vi "Interlock 32T Network Client.vi"() -> ()   [LabVIEW 2019]
doc: "Author: Scott Hannahs <sth@magnet.fsu.edu>\nCopyright 2018 Florida State University, All rights reserved."
uses:
  Interlock/SubVI/RT System Auth Level.ctl
  Interlock/SubVI/PS Action Control.ctl
  Interlock/SubVI/Interlock RT FPGA Status Info.ctl
  Interlock/SubVI/Interlock 32T FPGA Configure Parameters.ctl
  SubVIs/Interlock 32T Net Client Globals.vi
  TCP Functions/TCP Read Length and Value (STR).vi
  TCP Functions/TCP Read Length and Value (Array Str).vi
  <vilib>/Utility/miscctls.llb/LVRectTypeDef.ctl
  <vilib>/Utility/miscctls.llb/LVPointTypeDef.ctl
panel:
  in  "Clear Quench":bool
  in  "Slew rate [T/min]":dbl format="%.3g"
  out "Field [T]":dbl format="%.6g"
  in  "Setpoint [T]":dbl format="%.6g"
  in  "PS Action":T1=enum."Item 1"
  out "Version":string
  in  "Clear error":bool
  in  "Front Panel Tab":T2(tab)
  out "Crowbar Unlock Safe Curr LED":bool
  out "Crowbar":bool
  out "Quench Loop HI=ON":bool
  out "Crowbar LED":bool
  out "Close Switchbox 2":bool
  out "LTS Crowbar Status":bool
  out "HTS Crowbar Status":bool
  out "Crowbar Unlock Key":bool
  out "Ramp to Zero Button":bool
  out "Ramp to Zero Reset Button":bool
  out "Switchbox 2 Interlock":bool
  out "Switchbox 1 Interlock":bool
  out "LHe Level 2":dbl format="%.1f"
  out "LHe Level 1":dbl format="%.1f"
  out "Currents":dbl[][](graph)
  out "LHe Level":dbl[](array[slide]) scale=0.0..100.0
  out "Crowbar Unlock Gauge":dbl(knob) scale=0.0..60.0
  out "RT0 Fault Loop Timers":i16[](array[numeric])
  out "Secondary QD Time Constant":enum16{"2000 mS", "1000 mS", "200 mS", "50 mS"}(ring)
  out "HTS LEM Current":dbl format="%.5f"
  out "LTS LEM Current":dbl format="%.5f"
  out "HTS Shunt Current":dbl format="%.5f"
  out "Battery Ground Resistor V":dbl format="%.3f"
  out "Switchbox 2 Contator Out":dbl format="%.3f"
  out "Switchbox 1 Contator Out":dbl format="%.3f"
  out "Battery Voltage":dbl format="%.3f"
  out "Battery Monitory Alarm":bool
  out "Protection Logic Power Alarm":fxp<+/-,24,5> format="%.3g"
  out "Interlock RT Fault Counter":i16
  in  "Ramp To Zero Loop Time (mSec)":u32=40
  in  "PS-Disconnect Check Loop Time (mSec)":u32=40
  in  "Client Loop Time (mS)":u32=1000
  in  "Battery Low Warn":dbl format="%.1f"
  in  "Trip Threshold Currents":i16[](array[numeric])=[0, 50, 50]
  in  "Battery Voltage Scale":dbl=200.0
  in  "SW1 Vout Thresh":dbl=15.0
  in  "Quench Loop Thresh":dbl=1.5
  in  "# Low Readings":u32=3
  in  "Helium Low Level":dbl=3.0 format="%#_21g"
  in  "HTS LEM Scale":dbl=200.0
  in  "HTS Shunt Scale":dbl=40.0
  in  "LTS LEM Scale":dbl=360.0
  in  "Crowbar Loop Time (mSec)":u32=1
  in  "Interlock Check Loop Time (mSec)":u32=40
  in  "Main Loop Time (mSec)":u32=40
  in  "Turn Contactor OFF Current":dbl=1.0 format="%#_21g"
  in  "Turn Contactor ON Current":dbl=3.0 format="%#_21g"
  out "Start DateStamp":timestamp format="%<%H:%M:%S%4u\n%Y/%m/%d>T"
  out "Version RT System":string
  out "Version FPGA":string
  in  "Password":string
  in  "Save FPGA Config":bool
  in  "Read FPGA Config":bool
  out "Authorized":T3
  in  "HTS Shunt Offset (V)":dbl=40.0 format="%.4f"
  out "Download Progress":u8(slide) scale=0.0..100.0
  in  "File List":i32(listbox)=-1
  out "# Clients":u32
  out "# Timeout Err":u32
  out "Chassis Temperature":fxp<+/-,16,14> format="%.2g"
  out "Error Out":errorcluster
  in  "stop":bool
  # "NHMFL 32T\nInterlock"
  # "Indicators"
  # "Helium Levels"
  # "Coil Currents"
  # "Switch Box Status"
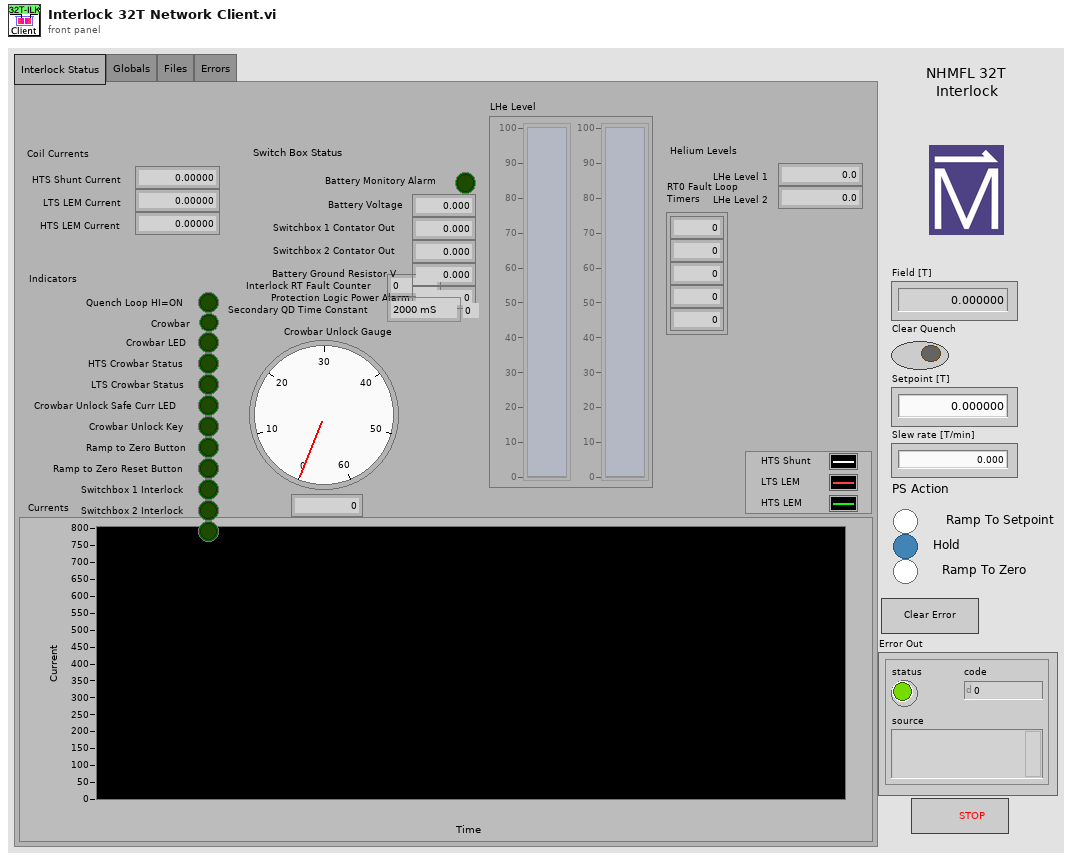
[diagram p1: front panel]
types:
  T1 = typedef "PS Action Control.ctl" = enum32{"Item 0", "Item 1", "Ramp To Zero"}
  T2 = enum32{"Interlock Status", "Globals", "Files", "Errors"}
  T3 = typedef "RT System Auth Level.ctl" = enum16{"Read Only", "User", "Operator", "Admin"}
  T4 = enum8{"Enabled", "Disabled", "Disabled and Grayed Out"}
  T5 = typedef "LVPointTypeDef.ctl" = cluster{"Horizontal":i16, "Vertical":i16}
  T6 = typedef "LVRectTypeDef.ctl" = cluster{"Left":i16, "Top":i16, "Right":i16, "Bottom":i16}
  T7 = enum16{"Standard", "Buffered", "CRLF", "Immediate"}
  T8 = typedef "Interlock 32T FPGA Configure Parameters.ctl" = cluster{"HTS LEM Scale":fxp<+/-,12,10>, "HTS Shunt Scale":fxp<+/-,16,14>, "LTS LEM Scale":fxp<+/-,12,10>, "Crowbar Loop Time (mSec)":u32, "Interlock Check Loop Time (mSec)":u32, "Main Loop Time (mSec)":u32, "Trip Threshold Currents":i16[], "Turn Contactor OFF Current":fxp<+/-,24,5>, "Turn Contactor ON Current":fxp<+/-,24,5>, "Helium Low Levels":dbl, "Quench Loop Thresh":fxp<+/-,24,5>, "SW1 Vout Thresh":fxp<+/-,24,5>, "Battery Voltage Scale":fxp<+/-,12,10>, "Battery Low Warn":dbl, "HTS Shunt Offset (V)":fxp<+/-,16,1>, "# Low Readings":u32, "PS-Disconnect Loop Time (mSec) ":u32, "Ramp To Zero Loop Time (mSec)":u32}
  T9 = typedef "Interlock RT FPGA Status Info.ctl" = cluster{"Authorized":T3, "# Clients":u32, "Chassis Temperature":fxp<+/-,16,14>, "Ramp To Zero":bool, "Crowbar":bool, "HTS Shunt":fxp<+/-,28,10>, "HTS LEM":fxp<+/-,36,15>, "LTS LEM":fxp<+/-,28,10>, "0 Reset Rt0 Button":bool, "2 Switchbox 2 Interlock":bool, "3 Switchbox 1 Interlock":bool, "5 Crowbar Unlock Safe Current LED":bool, "7 Crowbar LED":bool, "8 Ramp to Zero Button":bool, "13 Crowbar Unlock Key":bool, "15 Close Switch Box 2 Contactor":bool, "19 Battery monitor Alarm":bool, "Secondary QD Time Constant":enum16{"2000 mS", "1000 mS", "200 mS", "50 mS"}, "Loop timers":i16[], "Crowbar Latch State":i8, "Crowbar Reset Countdown Length (ms)":i32, "Crowbar Reset Countdown":i32, "Protection Petting Fault Counter":i16, "Watchdog Petting":bool, "Ramp to Zero Loop Fault Counter":i16, "Crowbar Loop Fault Counter":i16, "Main Loop Fault Counter":i16, "Interlock Petting":bool, "LTS Crowbar Status":bool, "HTS Crowbar Status":bool, "Battery Voltage":fxp<+/-,24,11>, "Protection Logic Power Alarm":fxp<+/-,24,5>, "Switchbox 2 Contactor Out":fxp<+/-,24,5>, "Battery ground resistor V":fxp<+/-,24,5>, "Switchbox 1 Contactor Out":fxp<+/-,24,5>, "Quench Loop":fxp<+/-,24,5>, "Quench Loop OK LED":bool, "10 Interlock RT Fault Counter":i16, "LHe Level 2":dbl, "LHe Level 1":dbl}
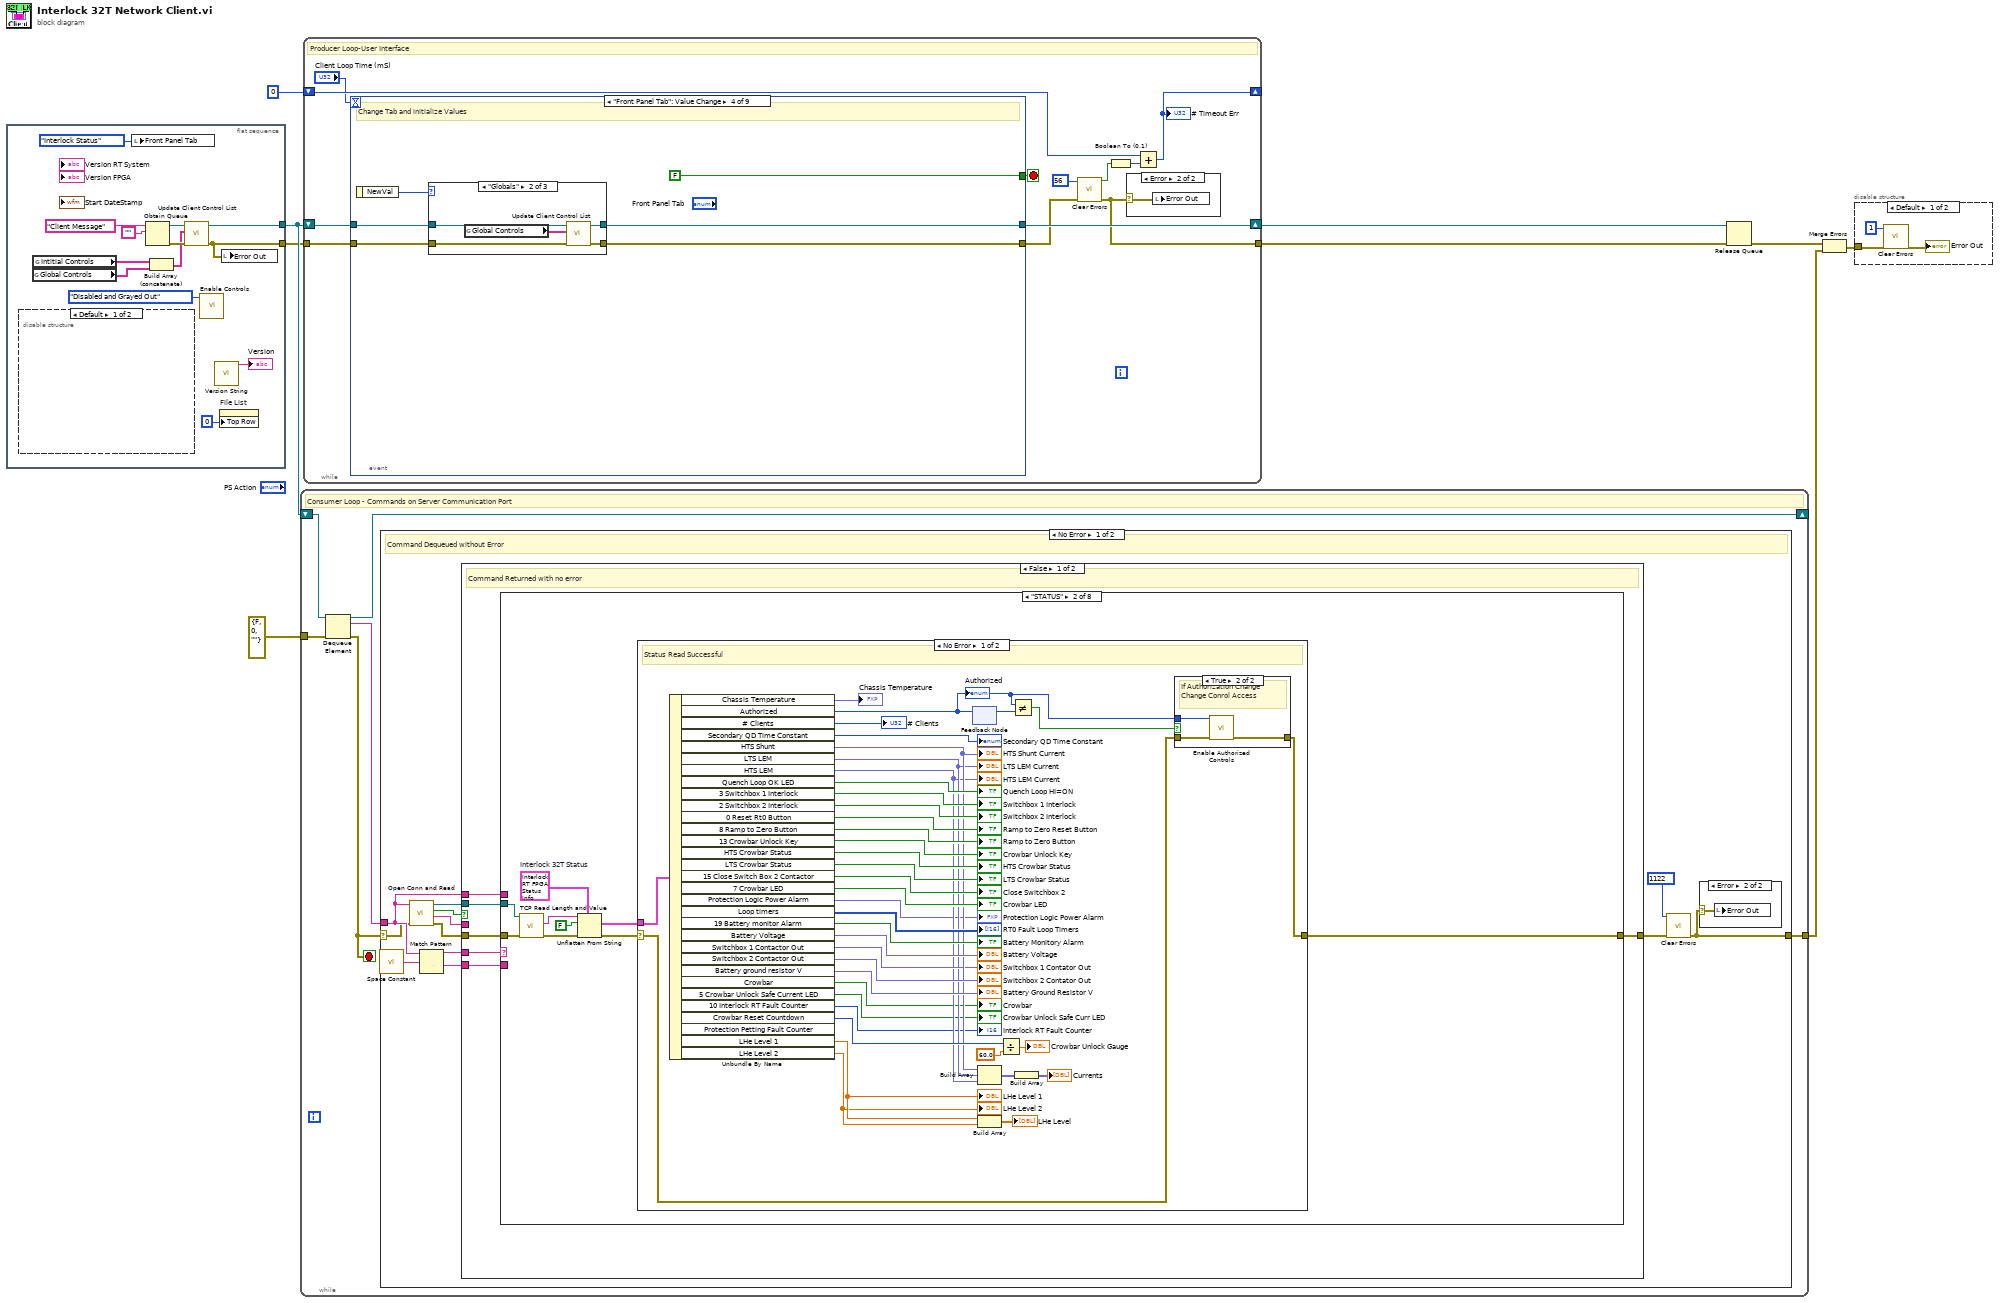
[diagram p0: block diagram]
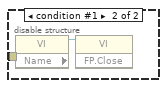
[diagram p2: hidden frame]
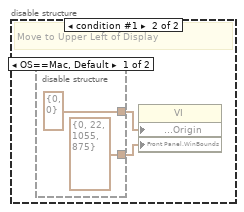
[diagram p3: hidden frame]
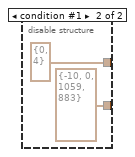
[diagram p4: hidden frame]
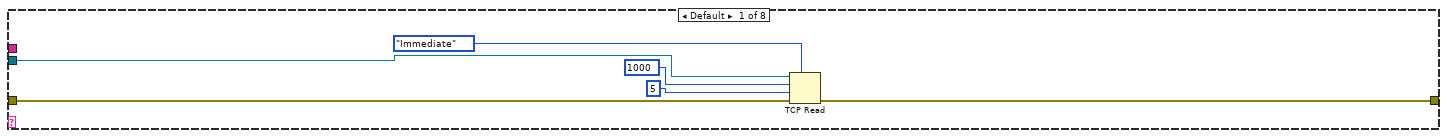
[diagram p6: hidden frame]
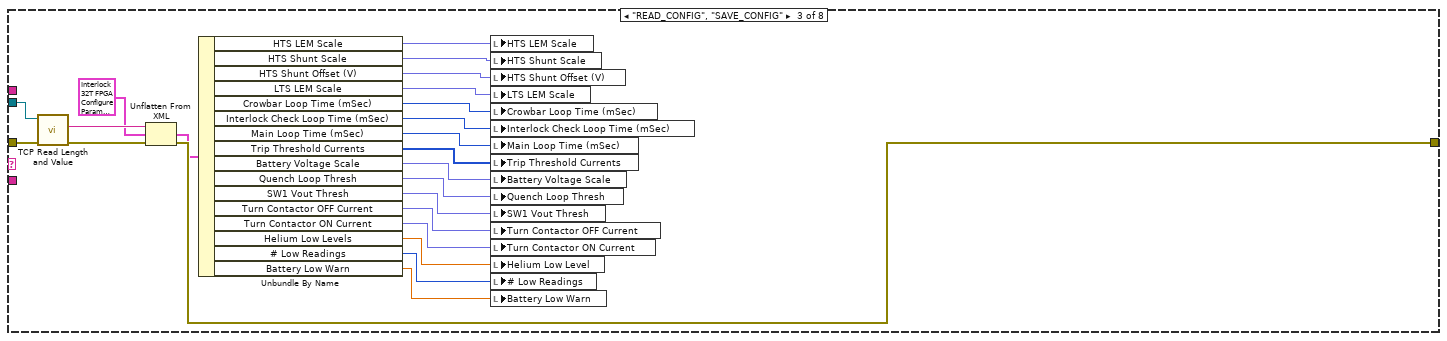
[diagram p9: hidden frame]
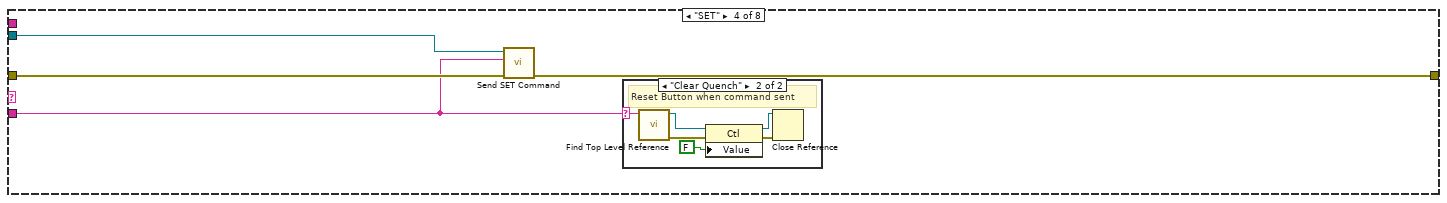
[diagram p10: hidden frame]
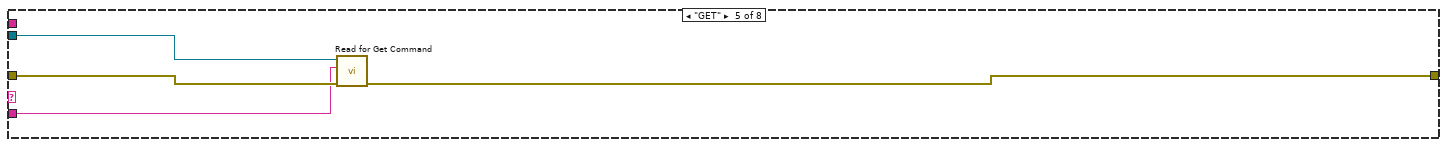
[diagram p12: hidden frame]
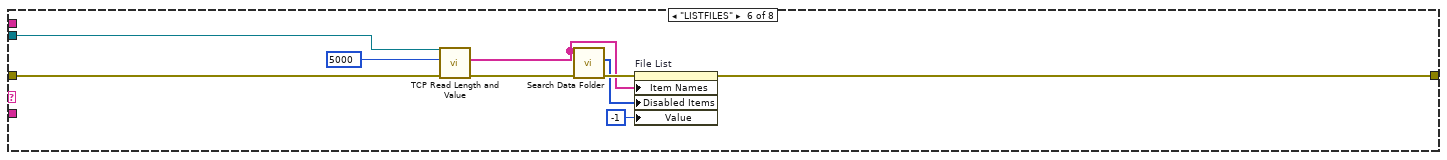
[diagram p13: hidden frame]
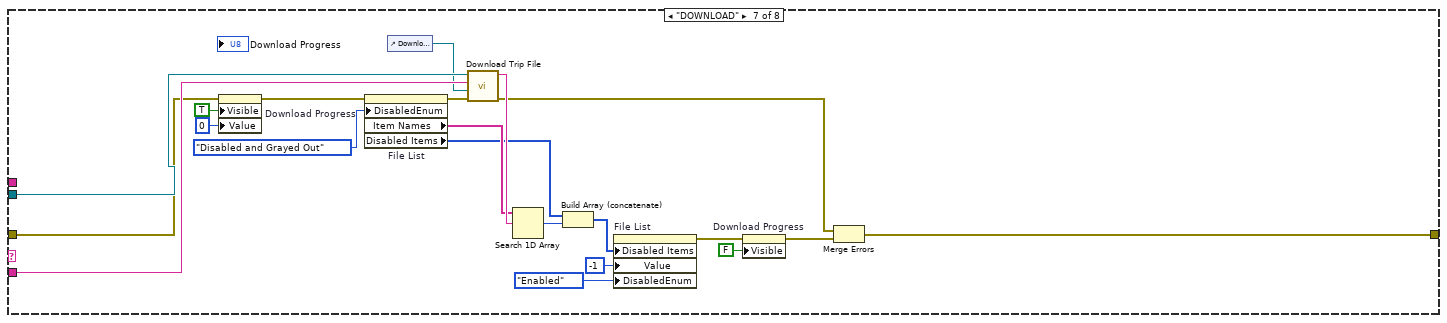
[diagram p14: hidden frame]
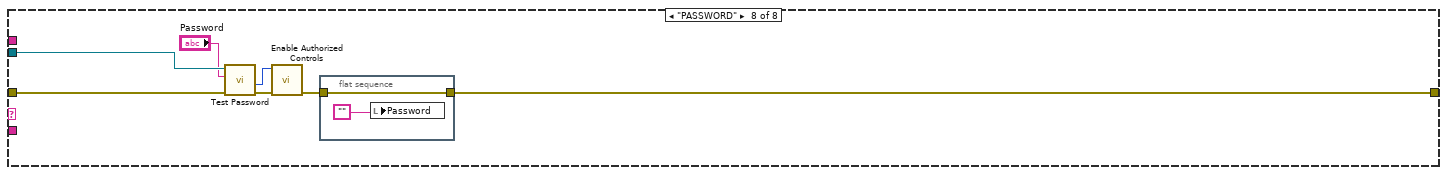
[diagram p15: hidden frame]
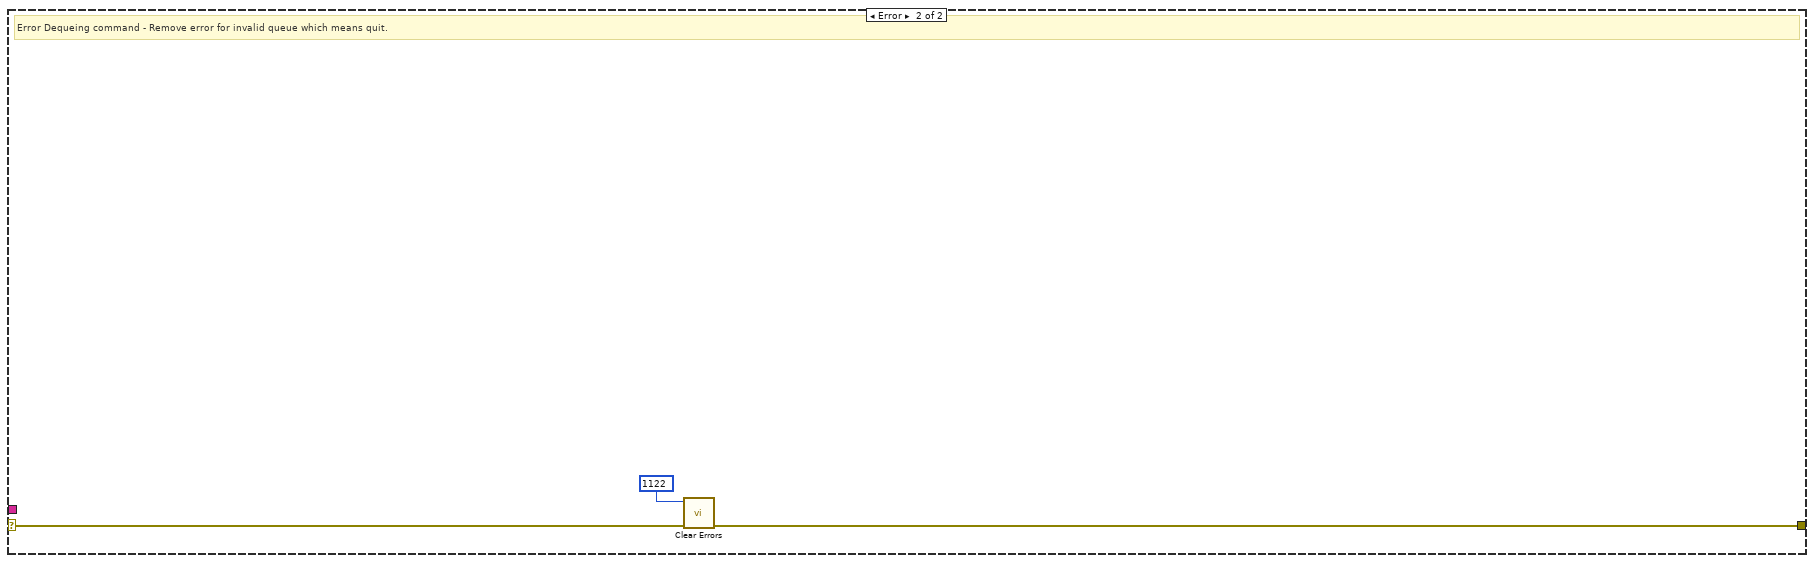
[diagram p17: hidden frame]
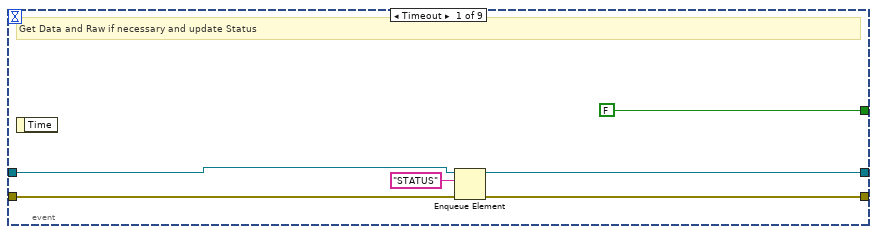
[diagram p19: hidden frame]
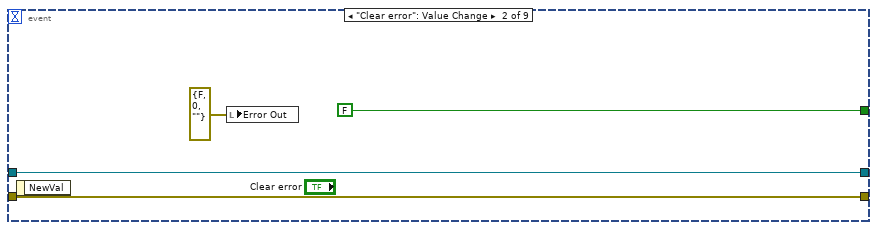
[diagram p20: hidden frame]
diagram:
  n1 = flat-sequence {
    tunnel: [w22] -> w5
    tunnel: [w17] -> w2
    frame #0 {
      n2 = disable-structure shown="Default" {
        frame condition #0 (active) {
        }
        frame condition #1 {
          # "Move to Upper Left of Display"
          n3 = disable-structure shown="OS==Mac, Default" {
            disable-tunnel: [T6 {"Left"=0, "Top"=22, "Right"=1055, "Bottom"=875} ("Front Panel Window:Window Bounds") T6 {"Left"=-10, "Top"=0, "Right"=1059, "Bottom"=883} ("Front Panel Window:Window Bounds")] -> w24
            disable-tunnel: [T5 {"Horizontal"=0, "Vertical"=0} ("Front Panel Window:Origin") T5 {"Horizontal"=0, "Vertical"=4} ("Front Panel Window:Origin")] -> w23
            frame condition #0 (active) {
            }
            frame condition #1 {
            }
          }
          n4 = property class="VI"("Front Panel Window:Origin"=w23, "Front Panel.WinBounds"=w24) -> ()  [unwired: 2 in, 2 out]
        }
      }
      n5 = global read "Interlock 32T Net Client Globals.vi" "Global Controls"() -> (w11:string[])
      n6 = global read "Interlock 32T Net Client Globals.vi" "Intitial Controls"() -> (w13:string[])
      n7 = local write "Front Panel Tab"(T2."Interlock Status" ("Front Panel Tab")) -> ()
      n8 = Obtain Queue(name (unnamed)="Client Message", element data type="") -> (queue out=w19:refnum<queue>, error out=w18:errorcluster)  [unwired: 3 in, 1 out]
      n9 = Build Array (concatenate)(w13, w11) -> (w15:string[])
      n10 = call "Update Client Control List.vi"("error in (no error)"=w18, "Array"=w15, "Queue in"=w19) -> ("error out"=w17:errorcluster, "Queue out"=w22:refnum<queue>)  [unwired: 7 in]
      n11 = call "Enable Controls.vi"("Enable Disable"=T4."Disabled and Grayed Out") -> ()  [unwired: 10 in, 1 out]
      n12 = call "Version String.vi"() -> ("String"=→"Version":string)  [unwired: 10 in, 1 out]
      n13 = property on="File List" class="LstBox (strict)"("Top Row"=0) -> ()  [unwired: 2 in, 2 out]
      n14 = local write "Error Out"(w17) -> ()
    }
  }
  n15 = while {
    shift-right: [w32] -> _
    shift-left: w5 -> [w34]
    tunnel: errorcluster {"status"=FALSE, "code"=0, "source"=""} ("error IO") -> [w33]
    tunnel: [w29] -> w3
    stop <- w30 stop-if-true
    # "Consumer Loop - Commands on Server Communication Port"
    n16 = Dequeue Element(queue=w34, error in (no error)=w33) -> (queue out=w32:refnum<queue>, element=w31:string, error out=w30:errorcluster)  [unwired: 1 in, 1 out]
    n17 = case shown="No Error" w30 {
      selector: w30 -> [w38 w193]
      tunnel: [w36 w192] -> w29
      tunnel: w31 -> [w42 _]
      frame No Error {
        # "Command Dequeued without Error"
        n18 = call <vilib>:"Space Constant.vi"() -> ("String"=w40:string)
        n19 = call "Open Conn and Read.vi"("error in (no error)"=w38, "String"=w42) -> ("error out"=w44:errorcluster, "Returned String"=w46:string, "Returned Error"=w43:bool, "TCP Network Connection out"=w45:refnum<k5>)  [unwired: 6 in]
        n20 = Match Pattern(string=w42, regular expression=w40) -> (before substring=w41:string, after substring=w39:string)  [unwired: 1 in, 2 out]
        n21 = case shown="False" w43 {
          tunnel: [w53 w190] -> w35
          tunnel: w46 -> [_ _]
          tunnel: w45 -> [w52 _]
          tunnel: w44 -> [w51 w190]
          tunnel: w42 -> [w50 _]
          tunnel: w41 -> [w49 _]
          tunnel: w39 -> [w48 _]
          frame False {
            # "Command Returned with no error"
            n22 = case shown="\"STATUS\"" w49 {
              tunnel: [w54 w60 w131 w139 w148 w153 w163 w184] -> w53
              tunnel: w51 -> [w56 w67 w135 w140 w149 w159 w170 w187]
              tunnel: w52 -> [w55 w66 w136 w138 w150 w158 w180 w186]
              tunnel: w50 -> [_ _ _ _ _ _ _ _]
              tunnel: w48 -> [_ _ _ w137 w147 _ w175 _]
              frame Default {
                n23 = TCP Read(connection ID=w55, bytes to read=1000, error in (no error)=w56, 7:T7."Immediate" ("mode (standard)"), 9:5 ("timeout ms (25000)")) -> (error out=w54:errorcluster)  [unwired: 2 out]
              }
              frame "STATUS" {
                w62 = T9 {"Authorized"=enum."Read Only", "# Clients"=0, "Chassis Temperature"=0.0, "Ramp To Zero"=FALSE, "Crowbar"=FALSE, "HTS Shunt"=0.0, "HTS LEM"=0.0, "LTS LEM"=0.0, "0 Reset Rt0 Button"=FALSE, "2 Switchbox 2 Interlock"=FALSE, "3 Switchbox 1 Interlock"=FALSE, "5 Crowbar Unlock Safe Current LED"=FALSE, "7 Crowbar LED"=FALSE, "8 Ramp to Zero Button"=FALSE, "13 Crowbar Unlock Key"=FALSE, "15 Close Switch Box 2 Contactor"=FALSE, "19 Battery monitor Alarm"=FALSE, "Secondary QD Time Constant"=enum."2000 mS", "Loop timers"=[0, 0, 0, 0, 0], "Crowbar Latch State"=0, "Crowbar Reset Countdown Length (ms)"=0, "Crowbar Reset Countdown"=0, "Protection Petting Fault Counter"=0, "Watchdog Petting"=FALSE, "Ramp to Zero Loop Fault Counter"=0, "Crowbar Loop Fault Counter"=0, "Main Loop Fault Counter"=0, "Interlock Petting"=FALSE, "LTS Crowbar Status"=FALSE, "HTS Crowbar Status"=FALSE, "Battery Voltage"=0.0, "Protection Logic Power Alarm"=0.0, "Switchbox 2 Contactor Out"=0.0, "Battery ground resistor V"=0.0, "Switchbox 1 Contactor Out"=0.0, "Quench Loop"=0.0, "Quench Loop OK LED"=FALSE, "10 Interlock RT Fault Counter"=0, "LHe Level 2"=3.334085464477539, "LHe Level 1"=2.148782730102539}  # Interlock 32T Status
                n24 = call-poly "TCP Read Length and Value.vi"("error in (no error)"=w67, "TCP Network Connection in"=w66) -> ("error out"=w68:errorcluster, "Output"=w64:string)  [unwired: 7 in, 1 out]
                n25 = Unflatten From String(type=w62, binary string=w64, data includes array or string size? (T)=FALSE, error in (no error)=w68) -> (value=w65:T9, error out=w61:errorcluster)  [unwired: 1 in, 1 out]
                n26 = case shown="No Error" w61 {
                  selector: w61 -> [w103 w113]
                  tunnel: w65 -> [w108 _]
                  tunnel: [w102 w113] -> w60
                  frame No Error {
                    # "Status Read Successful"
                    n27 = Unbundle By Name(w108) -> ("Chassis Temperature"=→"Chassis Temperature":fxp<+/-,16,14>, "Authorized"=w104:T3, "# Clients"=→"# Clients":u32, "Secondary QD Time Constant"=→"Secondary QD Time Constant":enum16{"2000 mS", "1000 mS", "200 mS", "50 mS"}, "HTS Shunt"=w79:fxp<+/-,28,10>, "LTS LEM"=w77:fxp<+/-,28,10>, "HTS LEM"=w76:fxp<+/-,36,15>, "Quench Loop OK LED"=→"Quench Loop HI=ON":bool, "3 Switchbox 1 Interlock"=→"Switchbox 1 Interlock":bool, "2 Switchbox 2 Interlock"=→"Switchbox 2 Interlock":bool, "0 Reset Rt0 Button"=→"Ramp to Zero Reset Button":bool, "8 Ramp to Zero Button"=→"Ramp to Zero Button":bool, "13 Crowbar Unlock Key"=→"Crowbar Unlock Key":bool, "HTS Crowbar Status"=→"HTS Crowbar Status":bool, "LTS Crowbar Status"=→"LTS Crowbar Status":bool, "15 Close Switch Box 2 Contactor"=→"Close Switchbox 2":bool, "7 Crowbar LED"=→"Crowbar LED":bool, "Protection Logic Power Alarm"=→"Protection Logic Power Alarm":fxp<+/-,24,5>, "Loop timers"=→"RT0 Fault Loop Timers":i16[], "19 Battery monitor Alarm"=→"Battery Monitory Alarm":bool, "Battery Voltage"=→"Battery Voltage":fxp<+/-,24,11>, "Switchbox 1 Contactor Out"=→"Switchbox 1 Contator Out":fxp<+/-,24,5>, "Switchbox 2 Contactor Out"=→"Switchbox 2 Contator Out":fxp<+/-,24,5>, "Battery ground resistor V"=→"Battery Ground Resistor V":fxp<+/-,24,5>, "Crowbar"=→"Crowbar":bool, "5 Crowbar Unlock Safe Current LED"=→"Crowbar Unlock Safe Curr LED":bool, "10 Interlock RT Fault Counter"=→"Interlock RT Fault Counter":i16, "Crowbar Reset Countdown"=w87:i32, "LHe Level 1"=w75:dbl, "LHe Level 2"=w74:dbl)  [unwired: 1 out]
                    "Authorized" <- w104
                    "HTS Shunt Current" <- w79
                    "LTS LEM Current" <- w77
                    "HTS LEM Current" <- w76
                    "LHe Level 1" <- w75
                    "LHe Level 2" <- w74
                    n28 = feedback-in #1(w104) -> ()
                    n29 = feedback #1() -> (w106:T3)  [unwired: 1 in]
                    n30 = Build Array(w79, w77, w76) -> (w81:fxp<+/-,36,15>[])
                    n31 = Build Array(w75, w74) -> (→"LHe Level":dbl[])
                    n32 = Divide(x=w87, y=60.0) -> (x/y=→"Crowbar Unlock Gauge":dbl)
                    n33 = Not Equal?(x=w104, y=w106) -> (x != y?=w105:bool)
                    n34 = Build Array(w81) -> (→"Currents":fxp<+/-,36,15>[][])
                    n35 = case shown="True" w105 {
                      tunnel: w104 -> [_ w112]
                      tunnel: w103 -> [w109 w111]
                      tunnel: [w109 w110] -> w102
                      frame False {
                      }
                      frame True {
                        # "If Authorization Change\nChange Conrol Access"
                        n36 = call "Enable Authorized Controls.vi"("error in (no error)"=w111, "Authorized"=w112) -> ("error out"=w110:errorcluster)  [unwired: 9 in]
                      }
                    }
                  }
                  frame Error {
                    # "Status Not Read"
                  }
                }
              }
              frame "READ_CONFIG", "SAVE_CONFIG" {
                n37 = call-poly "TCP Read Length and Value.vi"("error in (no error)"=w135, "TCP Network Connection in"=w136) -> ("error out"=w133:errorcluster, "Output"=w134:string)  [unwired: 7 in, 1 out]
                n38 = Unflatten From XML(xml string=w134, type=T8 {"HTS LEM Scale"=10.0, "HTS Shunt Scale"=511.75, "LTS LEM Scale"=0.25, "Crowbar Loop Time (mSec)"=4000000, "Interlock Check Loop Time (mSec)"=0, "Main Loop Time (mSec)"=0, "Trip Threshold Currents"=[0, 50, 50], "Turn Contactor OFF Current"=0.001953125, "Turn Contactor ON Current"=15.999998092651367, "Helium Low Levels"=3.0, "Quench Loop Thresh"=1.5, "SW1 Vout Thresh"=15.0, "Battery Voltage Scale"=200.0, "Battery Low Warn"=450.0, "HTS Shunt Offset (V)"=0.999969482421875, "# Low Readings"=3, "PS-Disconnect Loop Time (mSec) "=500, "Ramp To Zero Loop Time (mSec)"=10} ("Interlock 32T FPGA Configuration Values In"), error in (no error)=w133) -> (value=w130:T8, error out=w131:errorcluster)
                n39 = Unbundle By Name(w130) -> ("HTS LEM Scale"=w129:fxp<+/-,12,10>, "HTS Shunt Scale"=w128:fxp<+/-,16,14>, "HTS Shunt Offset (V)"=w114:fxp<+/-,16,1>, "LTS LEM Scale"=w127:fxp<+/-,12,10>, "Crowbar Loop Time (mSec)"=w126:u32, "Interlock Check Loop Time (mSec)"=w125:u32, "Main Loop Time (mSec)"=w124:u32, "Trip Threshold Currents"=w123:i16[], "Battery Voltage Scale"=w117:fxp<+/-,12,10>, "Quench Loop Thresh"=w118:fxp<+/-,24,5>, "SW1 Vout Thresh"=w119:fxp<+/-,24,5>, "Turn Contactor OFF Current"=w122:fxp<+/-,24,5>, "Turn Contactor ON Current"=w121:fxp<+/-,24,5>, "Helium Low Levels"=w120:dbl, "# Low Readings"=w116:u32, "Battery Low Warn"=w115:dbl)
                n40 = local write "HTS LEM Scale"(w129) -> ()
                n41 = local write "HTS Shunt Scale"(w128) -> ()
                n42 = local write "HTS Shunt Offset (V)"(w114) -> ()
                n43 = local write "LTS LEM Scale"(w127) -> ()
                n44 = local write "Crowbar Loop Time (mSec)"(w126) -> ()
                n45 = local write "Interlock Check Loop Time (mSec)"(w125) -> ()
                n46 = local write "Main Loop Time (mSec)"(w124) -> ()
                n47 = local write "Trip Threshold Currents"(w123) -> ()
                n48 = local write "Battery Voltage Scale"(w117) -> ()
                n49 = local write "Quench Loop Thresh"(w118) -> ()
                n50 = local write "SW1 Vout Thresh"(w119) -> ()
                n51 = local write "Turn Contactor OFF Current"(w122) -> ()
                n52 = local write "Turn Contactor ON Current"(w121) -> ()
                n53 = local write "Helium Low Level"(w120) -> ()
                n54 = local write "# Low Readings"(w116) -> ()
                n55 = local write "Battery Low Warn"(w115) -> ()
              }
              frame "SET" {
                n56 = call "Send SET Command.vi"("error in (no error)"=w140, "Control Name"=w137, "TCP Network Connection in"=w138) -> ("error out"=w139:errorcluster)  [unwired: 8 in]
                n57 = case shown="\"Clear Quench\"" w137 {
                  selector: w137 -> [_ w146]
                  frame Default {
                  }
                  frame "Clear Quench" {
                    # "Reset Button when command sent"
                    n58 = call "Find Top Level Reference.vi"("String"=w146) -> ("error out"=w141:errorcluster, "Ctl Refnum"=w145:refnum<vi>)  [unwired: 9 in]
                    n59 = property class="Ctl"(reference=w145, error in=w141, "Value"=FALSE) -> (reference out=w142:refnum<vi>, error out=w143:errorcluster)
                    n60 = Close Reference(reference=w142, error in (no error)=w143) -> ()  [unwired: 1 out]
                  }
                }
              }
              frame "GET" {
                n61 = call "Read for Get Command.vi"("error in (no error)"=w149, "Control Name"=w147, "TCP Network Connection in"=w150) -> ("error out"=w148:errorcluster)  [unwired: 8 in]
              }
              frame "LISTFILES" {
                n62 = call-poly "TCP Read Length and Value.vi"("error in (no error)"=w159, "timeout ms (1000)"=5000, "TCP Network Connection in"=w158) -> ("error out"=w157:errorcluster, "Output"=w154:string[])  [unwired: 6 in, 1 out]
                n63 = call "Search Data Folder.vi"("error in (no error)"=w157, "Server File List"=w154) -> ("error out"=w156:errorcluster, "Disabled Items"=w155:i32[])  [unwired: 8 in]
                n64 = property on="File List" class="LstBox (strict)"(error in=w156, "Item Names"=w154, "Disabled Items"=w155, "Value"=-1 ("File List")) -> (error out=w153:errorcluster)  [unwired: 1 in, 1 out]
              }
              frame "DOWNLOAD" {
                n65 = property on="Download Progress" class="Slide (strict)"(error in=w170, "Visible"=TRUE, "Value"=u8 0 ("Download Progress")) -> (error out=w165:errorcluster)  [unwired: 1 in, 1 out]
                n66 = property on="File List" class="LstBox (strict)"(error in=w165, "DisabledEnum"=T4."Disabled and Grayed Out" ("Disabled")) -> (error out=w164:errorcluster, "Item Names"=w161:string[], "Disabled Items"=w160:i32[])  [unwired: 1 in, 1 out]
                n67 = control-ref of="Download Progress"() -> (w172:refnum<vi>)
                n68 = call "Download Trip File.vi"("error in (no error)"=w164, "Download Progress Ref"=w172, "File Name"=w175, "TCP Network Connection in"=w180) -> ("error out"=w162:errorcluster, "File Name Out"=w177:string)  [unwired: 6 in]
                n69 = Search 1D Array(1D array=w161, element=w177) -> (index of element=w178:i32)  [unwired: 1 in]
                n70 = Build Array (concatenate)(w160, w178) -> (w179:i32[])
                n71 = property on="File List" class="LstBox (strict)"("Disabled Items"=w179, "Value"=-1 ("File List"), "DisabledEnum"=T4."Enabled" ("Disabled")) -> (error out=w169:errorcluster)  [unwired: 2 in, 1 out]
                n72 = property on="Download Progress" class="Slide (strict)"(error in=w169, "Visible"=FALSE) -> (error out=w168:errorcluster)  [unwired: 1 in, 1 out]
                n73 = Merge Errors(w162, w168) -> (w163:errorcluster)
              }
              frame "PASSWORD" {
                n74 = call "Test Password.vi"("error in (no error)"=w187, "String"="Password", "TCP Network Connection in"=w186) -> ("error out"=w181:errorcluster, "Authorized"=w183:T3)  [unwired: 6 in, 1 out]
                n75 = call "Enable Authorized Controls.vi"("error in (no error)"=w181, "Authorized"=w183) -> ("error out"=w182:errorcluster)  [unwired: 9 in]
                n76 = flat-sequence {
                  tunnel: w182 -> [w189]
                  tunnel: [w189] -> w184
                  frame #0 {
                    n77 = local write "Password"("") -> ()
                  }
                }
              }
            }
          }
          frame True {
          }
        }
        n78 = call <vilib>:"Clear Errors.vi"("error in (no error)"=w35, "specific error code to clear (0: all)"=1122) -> ("error out"=w36:errorcluster)  [unwired: 4 in, 1 out]
        n79 = case shown="Error" w36 {
          selector: w36 -> [_ w47]
          frame No Error {
          }
          frame Error {
            n80 = local write "Error Out"(w47) -> ()
          }
        }
      }
      frame Error {
        # "Error Dequeing command - Remove error for invalid queue which means quit."
        n81 = call <vilib>:"Clear Errors.vi"("error in (no error)"=w193, "specific error code to clear (0: all)"=1122) -> ("error out"=w192:errorcluster)  [unwired: 4 in, 1 out]
      }
    }
  }
  n82 = while {
    tunnel: w2 -> [w195]
    tunnel: [w196] -> w4
    shift-right: [w203] -> _
    shift-left: u32 0 -> [w201]
    shift-right: [w199] -> w7
    shift-left: w5 -> [w200]
    stop <- w197 stop-if-true
    # "Producer Loop-User Interface"
    n83 = event shown="[3] \"Front Panel Tab\": Value Change" {
      selector: _ -> [_ _ _ _ _ _ _ _ _]
      dyn-events: _ -> [_ _ _ _ _ _ _ _ _]
      timeout: "Client Loop Time (mS)" -> [_ _ _ _ _ _ _ _ _]
      tunnel: w195 -> [w211 w214 w219 w224 w242 w252 w258 w268 w275]
      tunnel: [w207 w214 w219 w223 w240 w251 w257 w262 w274] -> w198
      tunnel: [w208 w215 w218 w222 w239 w250 w256 w261 w273] -> w199
      tunnel: w200 -> [w212 w215 w218 w221 w243 w253 w259 w264 w276]
      tunnel: [FALSE ("NewVal") FALSE ("NewVal") w217 FALSE ("NewVal") FALSE ("NewVal") FALSE ("NewVal") FALSE ("NewVal") FALSE ("NewVal") FALSE ("NewVal")] -> w197
      event Timeout {
        # "Get Data and Raw if necessary and update Status"
        n84 = event-data() -> ()  [unwired: 1 in, 1 out]
        n85 = Enqueue Element(queue=w212, element="STATUS", error in (no error)=w211) -> (queue out=w208:refnum<queue>, error out=w207:errorcluster)  [unwired: 1 in, 1 out]
      }
      event "Clear error": Value Change {
        n86 = event-data() -> ()  [unwired: 1 in, 1 out]
        n87 = local write "Error Out"(errorcluster {"status"=FALSE, "code"=0, "source"=""} ("Error Out")) -> ()
      }
      event "stop": Value Change {
        n88 = event-data() -> ("NewVal"=w217:bool)  [unwired: 1 in]
      }
      event "Front Panel Tab": Value Change {
        # "Change Tab and initialize Values"
        n89 = event-data() -> ("NewVal"=w225:T2)  [unwired: 1 in]
        n90 = case shown="\"Globals\"" w225 {
          tunnel: w224 -> [w226 w232 w234]
          tunnel: [w226 w231 w236] -> w223
          tunnel: [w227 w230 w237] -> w222
          tunnel: w221 -> [w227 w229 w235]
          frame "Errors", Default {
          }
          frame "Globals" {
            n91 = global read "Interlock 32T Net Client Globals.vi" "Global Controls"() -> (w228:string[])
            n92 = call "Update Client Control List.vi"("error in (no error)"=w232, "Array"=w228, "Queue in"=w229) -> ("error out"=w231:errorcluster, "Queue out"=w230:refnum<queue>)  [unwired: 7 in]
          }
          frame "Files" {
            n93 = Enqueue Element(queue=w235, element="ListFiles", error in (no error)=w234) -> (queue out=w237:refnum<queue>, error out=w236:errorcluster)  [unwired: 1 in, 1 out]
          }
        }
      }
      event "Turn Contactor ON Current", "Turn Contactor OFF Current", "Main Loop Time (mSec)", "Interlock Check Loop Time (mSec)", "Crowbar Loop Time (mSec)", "LTS LEM Scale", "HTS Shunt Scale", "HTS LEM Scale", "Helium Low Level", "Quench Loop Thresh", "SW1 Vout Thresh", "Battery Voltage Scale", "# Low Readings", "Trip Threshold Currents", "Clear Quench", "HTS Shunt Offset (V)", "Battery Low Warn", "PS-Disconnect Check Loop Time (mSec)", "Ramp To Zero Loop Time (mSec)": Value Change {
        # "Update Values on target"
        n94 = event-data() -> ("CtlRef"=w247:refnum<vi>)  [unwired: 1 in]
        n95 = property class="Ctl"(reference=w247, error in=w242) -> (error out=w245:errorcluster, "Label.Text"=w241:string)  [unwired: 1 out]
        n96 = Concatenate Strings("SET " ("string"), w241) -> (w244:string)
        n97 = Enqueue Element(queue=w243, element=w244, error in (no error)=w245) -> (queue out=w239:refnum<queue>, error out=w240:errorcluster)  [unwired: 1 in, 1 out]
      }
      event "Read FPGA Config": Value Change {
        n98 = event-data() -> ()  [unwired: 1 in, 1 out]
        n99 = Enqueue Element(queue=w253, element="Read_Config", error in (no error)=w252) -> (queue out=w250:refnum<queue>, error out=w251:errorcluster)  [unwired: 1 in, 1 out]
      }
      event "Save FPGA Config": Value Change {
        n100 = event-data() -> ()  [unwired: 1 in, 1 out]
        n101 = Enqueue Element(queue=w259, element="Save_Config", error in (no error)=w258) -> (queue out=w256:refnum<queue>, error out=w257:errorcluster)  [unwired: 1 in, 1 out]
      }
      event "File List": Value Change {
        n102 = event-data() -> ("NewVal"=w270:i32)  [unwired: 1 in]
        n103 = property on="File List" class="LstBox (strict)"(error in=w268) -> (error out=w263:errorcluster, "Item Names"=w269:string[])  [unwired: 1 in, 1 out]
        n104 = Index Array(array=w269, index=w270) -> (element=w267:string)
        n105 = Concatenate Strings("DOWNLOAD " ("string"), w267) -> (w265:string)
        n106 = Enqueue Element(queue=w264, element=w265, error in (no error)=w263) -> (queue out=w261:refnum<queue>, error out=w262:errorcluster)  [unwired: 1 in, 1 out]
      }
      event "Password": Value Change {
        n107 = event-data() -> ()  [unwired: 1 in, 6 out]
        n108 = Enqueue Element(queue=w276, element="PASSWORD" ("string"), error in (no error)=w275) -> (queue out=w273:refnum<queue>, error out=w274:errorcluster)  [unwired: 1 in, 1 out]
      }
    }
    n109 = call <vilib>:"Clear Errors.vi"("error in (no error)"=w198, "specific error code to clear (0: all)"=56) -> ("error out"=w196:errorcluster, "specific error cleared?"=w202:bool)  [unwired: 4 in]
    n110 = Boolean To (0,1)(Boolean=w202) -> (0, 1=w204:i16)
    n111 = case shown="Error" w196 {
      selector: w196 -> [_ w206]
      frame No Error {
      }
      frame Error {
        n112 = local write "Error Out"(w206) -> ()
      }
    }
    n113 = Add(x=w201, y=w204) -> (x+y=w203:u32)
    "# Timeout Err" <- w203
  }
  n114 = Release Queue(queue=w7, error in (no error)=w4) -> (error out=w6:errorcluster)  [unwired: 1 in, 2 out]
  n115 = Merge Errors(w6, w3) -> (w1:errorcluster)
  n116 = disable-structure shown="Default" {
    disable-tunnel: w1 -> [w279 _]
    frame condition #0 (active) {
      n117 = call <vilib>:"Clear Errors.vi"("error in (no error)"=w279, "specific error code to clear (0: all)"=1) -> ("error out"=→"Error Out":errorcluster)  [unwired: 4 in, 1 out]
    }
    frame condition #1 {
      n118 = property class="VI" props=["Name"]() -> (reference out=w280:refnum<vi>)  [unwired: 2 in, 2 out]
      n119 = invoke class="VI" method="FP.Close"(reference=w280) -> ()  [unwired: 2 in, 3 out]
    }
  }
